vi "Delay.vi"(8 "error in (no error)":errorcluster, 9 "milliseconds to wait":dbl=300.0 min=0.0 max=1000.0 format="%.3f") -> (0 "error out":errorcluster)   [LabVIEW 2015]
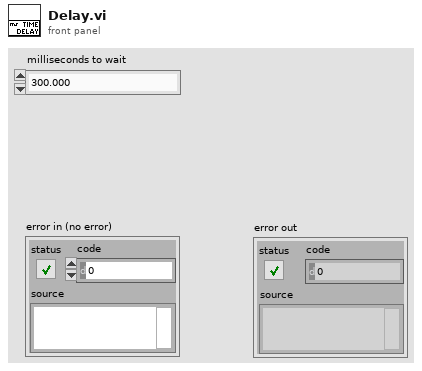
[diagram p1: front panel]
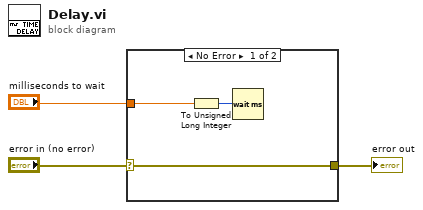
[diagram p0: block diagram]
diagram:
  n1 = case shown="No Error" "error in (no error)" {
    selector: "error in (no error)" -> [w6 w7]
    tunnel: [w6 w7] -> w3
    tunnel: "milliseconds to wait" -> [w4 _]
    frame No Error {
      n2 = To Unsigned Long Integer(number=w4) -> (unsigned 32bit integer=w5:u32)
      n3 = Wait (ms)(milliseconds to wait=w5) -> ()  [unwired: 1 out]
    }
    frame Error {
    }
  }
  "error out" <- w3
